vi "second state selector.vi"(8 "error in":errorcluster, 10 "state":T2=enum."Setup", 11 "Controls":T1) -> (0 "error out":errorcluster, 3 "state out":T2)   [LabVIEW 2015]
uses:
  controls/state.ctl
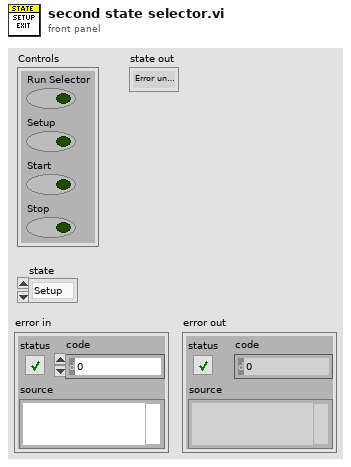
[diagram p1: front panel]
types:
  T1 = cluster{"Run Selector":bool, "Setup":bool, "Start":bool, "Stop":bool}
  T2 = typedef "state.ctl" = enum16{"Error under range", "Exit", "Initialize", "Start", "Error", "Run", "Setup", "Low pressure", "Rain", "Idle"}
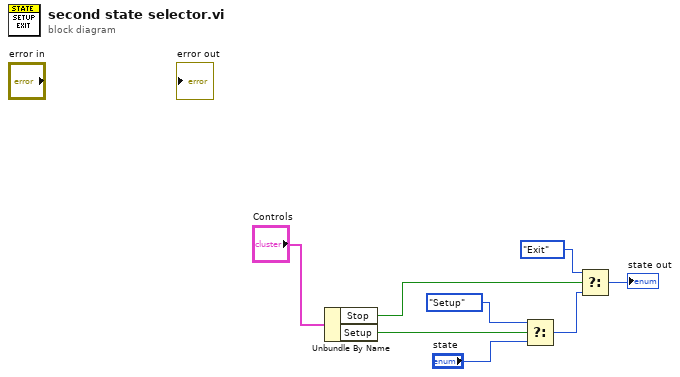
[diagram p0: block diagram]
diagram:
  n1 = Unbundle By Name("Controls") -> ("Stop"=w5:bool, "Setup"=w2:bool)
  n2 = Select(t=state."Setup" ("element"), s=w2, f="state") -> (s? t:f=w6:T2)
  n3 = Select(t=state."Exit", s=w5, f=w6) -> (s? t:f=→"state out":T2)
